vi "_interfacebrowser Build Interface Menu.vi"(5 "Tree":refnum<vi>, 7 "CtlRef":refnum<vi>, 9 "Coords":T1, 11 "Menu in":refnum<k9>) -> (3 "Discard?":bool)   [LabVIEW 2017]
uses:
  <vilib>/Utility/miscctls.llb/LVPoint32TypeDef.ctl
  Communicable State Machine.lvlib
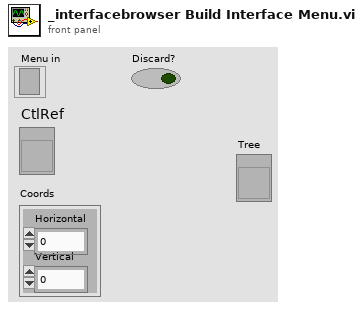
[diagram p1: front panel]
types:
  T1 = typedef "LVPoint32TypeDef.ctl" = cluster{"Horizontal":i32, "Vertical":i32}
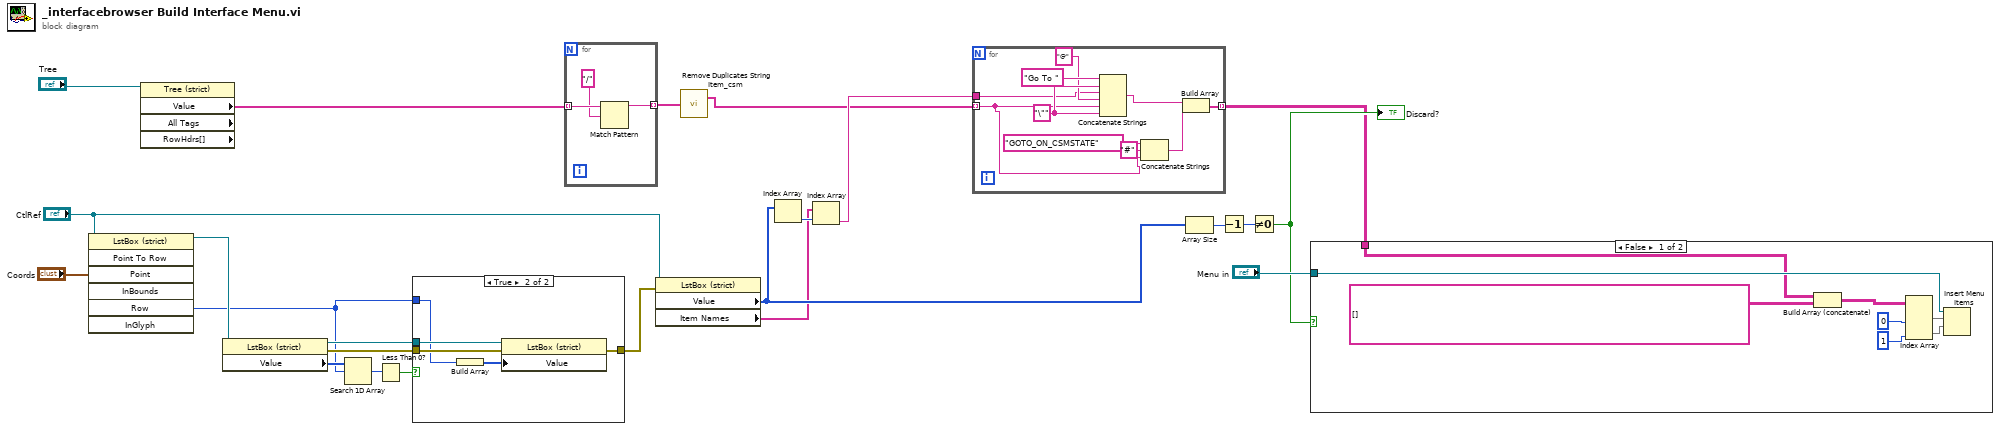
[diagram p0: block diagram]
diagram:
  n1 = invoke on="Invoke Node" class="LstBox (strict)" method="Point To Row"(reference="CtlRef", "Point"="Coords") -> (reference out=w18:refnum<vi>, "Row"=w11:i32)  [unwired: 5 in, 5 out]
  n2 = property on="Property Node" class="Tree (strict)" props=["Value", "All Tags", "RowHdrs[]"](reference="Tree") -> ("Value"=w3:string[])  [unwired: 1 in, 4 out]
  n3 = property on="Property Node" class="LstBox (strict)"(reference=w18) -> (reference out=w15:refnum<vi>, error out=w16:errorcluster, "Value"=w12:i32[])  [unwired: 1 in]
  n4 = Search 1D Array(1D array=w12, element=w11) -> (index of element=w17:i32)  [unwired: 1 in]
  n5 = Less Than 0?(x=w17) -> (x < 0?=w14:bool)
  n6 = case shown="True" w14 {
    tunnel: w16 -> [w24 w29]
    tunnel: w15 -> [_ w28]
    tunnel: w11 -> [_ w27]
    tunnel: [w24 w26] -> w13
    frame False {
    }
    frame True {
      n7 = Build Array(w27) -> (w25:i32[])
      n8 = property on="Property Node" class="LstBox (strict)"(reference=w28, error in=w29, "Value"=w25) -> (error out=w26:errorcluster)  [unwired: 1 out]
    }
  }
  n9 = for {
    tunnel: w3 -> [w32] mode=indexing
    tunnel: [w30] -> w2 mode=indexing
    n10 = Match Pattern(string=w32, regular expression="/") -> (before substring=w30:string)  [unwired: 1 in, 3 out]
  }
  n11 = property on="Property Node" class="LstBox (strict)"(reference="CtlRef", error in=w13) -> ("Value"=w7:i32[], "Item Names"=w5:string[])  [unwired: 2 out]
  n12 = call "Remove Duplicates String Item_csm.vi"("Input Array"=w2) -> ("Output Array"=w1:string[])  [unwired: 1 out]
  n13 = Index Array(array=w7) -> (element=w6:i32)  [unwired: 1 in]
  n14 = Index Array(array=w5, index=w6) -> (element=w4:string)
  n15 = for {
    tunnel: w1 -> [w33] mode=indexing
    tunnel: [w38] -> w8 mode=indexing
    tunnel: w4 -> [w36]
    w41 = "\"" ("string")
    n16 = Concatenate Strings("Go To " ("string"), w41, w36, "@" ("string"), w33, w41) -> (w40:string)
    n17 = Concatenate Strings("GOTO_ON_CSMSTATE", "#" ("string"), w33) -> (w35:string)
    n18 = Build Array(w40, w35) -> (w38:string[])
  }
  n19 = Array Size(array=w7) -> (size(s)=w19:i32)
  n20 = Decrement(x=w19) -> (x-1=w20:i32)
  n21 = Not Equal To 0?(x=w20) -> (x != 0?=w10:bool)
  "Discard?" <- w10
  n22 = case shown="False" w10 {
    tunnel: "Menu in" -> [w50 _]
    tunnel: w8 -> [w43 _]
    frame False {
      n23 = Build Array (concatenate)(w43, string[][] [] ("item names")) -> (w44:string[][])
      n24 = Index Array(array=w44, index (col) #1=0 ("disabled index (col)"), index (col) #2=1 ("index (col)")) -> (element #1=w48:string[], element #2=w47:string[])  [unwired: 2 in]
      n25 = Insert Menu Items(7:w47, 8:w48, 9:w50) -> ()  [unwired: 3 in, 3 out]
    }
    frame True {
    }
  }
